vi "Initialize Monitor Setting.vi"(7 "Channel number":i32=4, 8 "XY Graph REF":refnum<vi>, 11 "plot setting":refnum<vi>) -> ()   [LabVIEW 2023]
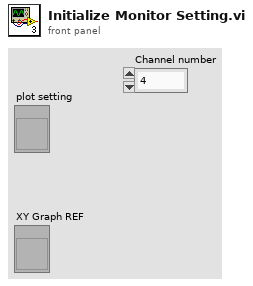
[diagram p1: front panel]
types:
  T1 = cluster{bool, "Plot.Visible":bool, "Plot.Plot Color":u32, string}
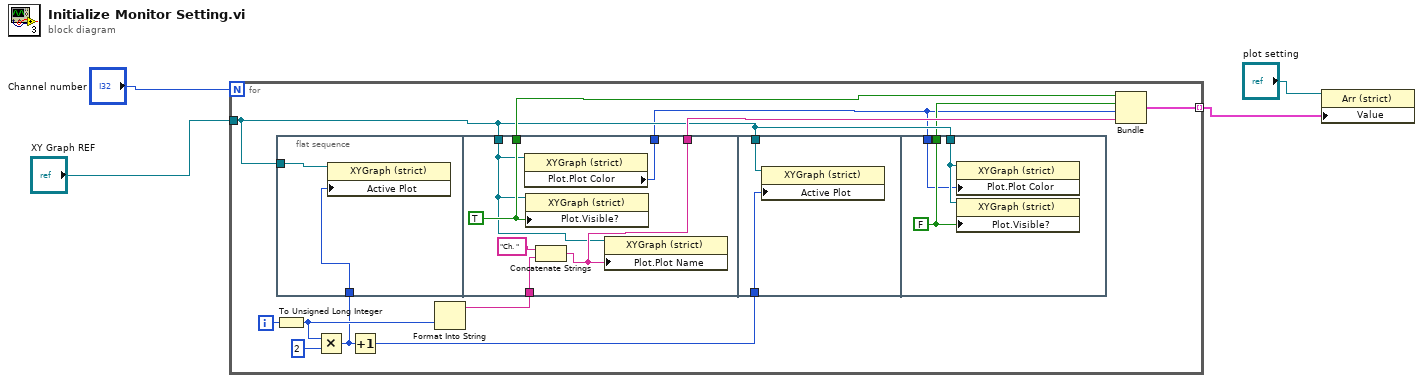
[diagram p0: block diagram]
diagram:
  n1 = for {
    N: "Channel number" -> [_]
    tunnel: "XY Graph REF" -> [w12]
    tunnel: [w10] -> w2 mode=indexing
    i -> [w15]
    n2 = To Unsigned Long Integer(number=w15) -> (unsigned 32bit integer=w8:u32)
    n3 = flat-sequence {
      tunnel: w12 -> [w18]
      tunnel: w5 -> [w17]
      tunnel: [w24] -> w16
      tunnel: [w23] -> w9
      tunnel: w14 -> [w21]
      tunnel: [w20] -> w13
      tunnel: w12 -> [w19]
      tunnel: w12 -> [w26]
      tunnel: w6 -> [w25]
      tunnel: w12 -> [w29]
      tunnel: [w28] -> w11
      tunnel: w9 -> [w27]
      frame #0 {
        n4 = property class="XYGraph (strict)"(reference=w18, "Active Plot"=w17) -> ()  [unwired: 1 in, 2 out]
      }
      frame #1 {
        w24 = TRUE
        n5 = property class="XYGraph (strict)"(reference=w19) -> ("Plot.Plot Color"=w23:u32)  [unwired: 1 in, 2 out]
        n6 = property class="XYGraph (strict)"(reference=w19, "Plot.Visible?"=w24) -> ()  [unwired: 1 in, 2 out]
        n7 = Concatenate Strings("Ch. " ("string"), w21) -> (w20:string)
        n8 = property class="XYGraph (strict)"(reference=w19, "Plot.Plot Name"=w20) -> ()  [unwired: 1 in, 2 out]
      }
      frame #2 {
        n9 = property class="XYGraph (strict)"(reference=w26, "Active Plot"=w25) -> ()  [unwired: 1 in, 2 out]
      }
      frame #3 {
        w28 = FALSE ("Plot.Visible")
        n10 = property class="XYGraph (strict)"(reference=w29, "Plot.Plot Color"=w27) -> ()  [unwired: 1 in, 2 out]
        n11 = property class="XYGraph (strict)"(reference=w29, "Plot.Visible?"=w28) -> ()  [unwired: 1 in, 2 out]
      }
    }
    n12 = Multiply(x=w8, y=u32 2) -> (x*y=w5:u32)
    n13 = Increment(x=w5) -> (x+1=w6:u32)
    n14 = Format Into String(w8) -> (resulting string=w14:string)  [unwired: 3 in, 1 out]
    n15 = Bundle(w16, "Plot.Visible"=w11, "Plot.Plot Color"=w9, w13) -> (w10:T1)  [unwired: 1 in]
  }
  n16 = property class="Arr (strict)"(reference="plot setting", "Value"=w2) -> ()  [unwired: 1 in, 2 out]
